vi "Loop Timer [Data Dependency].vi"() -> ()   [LabVIEW 2017]
panel:
  out "While Loop Time (ms)":u32
  out "For Loop Time (ms)":u32
  out "While Loop Array":i32[](array[numeric])
  out "For Loop Array":i32[](array[numeric])
  in  "Number of Elements":i32=10000000
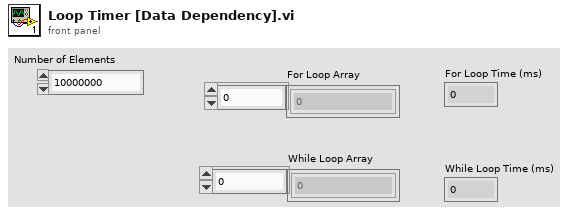
[diagram p1: front panel]
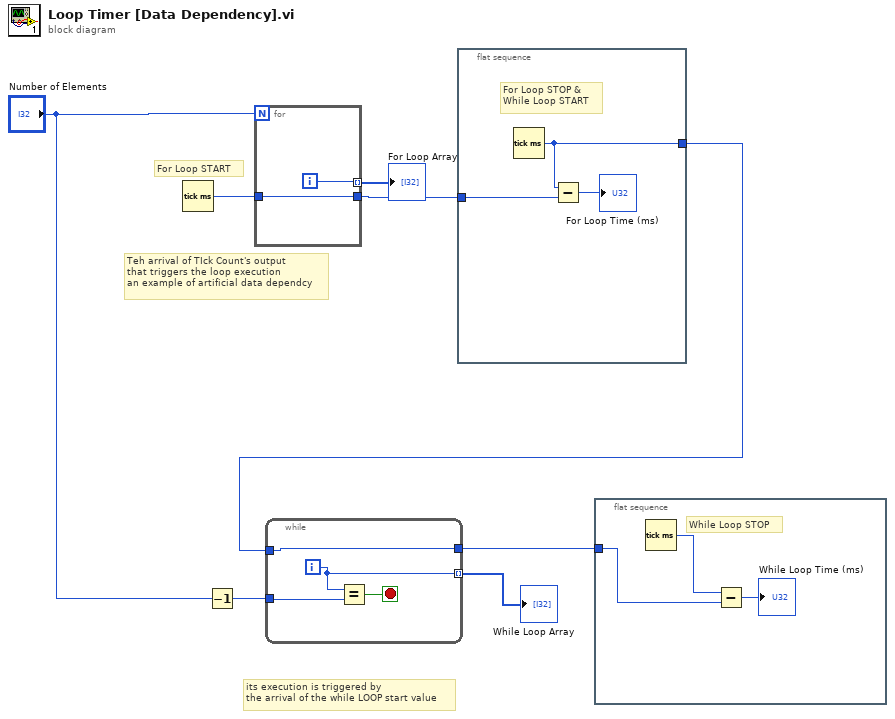
[diagram p0: block diagram]
diagram:
  # "its execution is triggered by \nthe arrival of the while LOOP start value"
  # "Teh arrival of TIck Count's output \nthat triggers the loop execution\nan example of artificial data dependcy"
  # "For Loop START"
  n1 = Tick Count (ms)() -> (millisecond timer value=w3:u32)
  n2 = Decrement(x="Number of Elements") -> (x-1=w8:i32)
  n3 = for {
    N: "Number of Elements" -> [_]
    tunnel: [w10] -> w7 mode=indexing
    tunnel: w3 -> [w9]
    tunnel: [w9] -> w5
    i -> [w10]
  }
  "For Loop Array" <- w7
  n4 = while {
    tunnel: w8 -> [w13]
    tunnel: [w12] -> w6 mode=indexing
    tunnel: w4 -> [w11]
    tunnel: [w11] -> w2
    i -> [w12]
    stop <- w14 stop-if-true
    n5 = Equal?(x=w12, y=w13) -> (x = y?=w14:bool)
  }
  "While Loop Array" <- w6
  n6 = flat-sequence {
    tunnel: [w16] -> w4
    tunnel: w5 -> [w15]
    frame #0 {
      # "For Loop STOP &\nWhile Loop START"
      n7 = Tick Count (ms)() -> (millisecond timer value=w16:u32)
      n8 = Subtract(x=w16, y=w15) -> (x-y=→"For Loop Time (ms)":u32)
    }
  }
  n9 = flat-sequence {
    tunnel: w2 -> [w18]
    frame #0 {
      # "While Loop STOP"
      n10 = Tick Count (ms)() -> (millisecond timer value=w19:u32)
      n11 = Subtract(x=w19, y=w18) -> (x-y=→"While Loop Time (ms)":u32)
    }
  }
